vi "GetErrorsOfLibrary.vi"(8 "ErrorIn":errorcluster caption="Error In(no Error)", 9 "LibraryName":string, 11 "ReferenceIn":refnum<class "ErrorDefinitionSQLite.lvclass"> caption="Reference In") -> (0 "ErrorOut":errorcluster caption="Error Out", 1 "Errors":T1, 3 "ReferenceOut":refnum<class "ErrorDefinitionSQLite.lvclass"> caption="Reference Out")   [LabVIEW 2018, in "ErrorDefinitionSQLite.lvclass"]
uses:
  <userlib>/_express/CustomErrorCreator/ErrorDefinitionSQLite/ErrorDefinitionSQLite.lvclass
  <userlib>/_express/CustomErrorCreator/ErrorDefinitionSQLite/ErrorContent.ctl
  <vilib>/drjdpowell/SQLite Library/SQL Connection/Open (path).vi
  <vilib>/drjdpowell/SQLite Library/SQL Connection/Open (string).vi
  <vilib>/AdvancedString/Path To Command Line String.vi
  <vilib>/drjdpowell/SQLite Library/SQL Connection/Execute SQL.vi
  <vilib>/drjdpowell/SQLite Library/SQL Connection/Connection.lvclass
  <vilib>/drjdpowell/SQLite Library/SQLite.lvlib
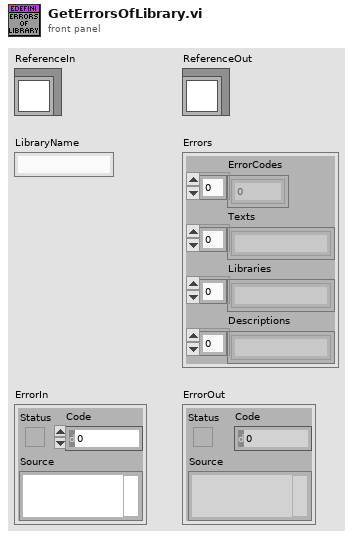
[diagram p1: front panel]
types:
  T1 = typedef "ErrorDefinitionSQLite.lvclass/ErrorContent.ctl" = cluster{"ErrorCodes":i32[], "Texts":string[], "Libraries":string[], "Descriptions":string[]}
  T2 = enum16{"New or existing", "Existing", "Read only"}
  T3 = typedef "ErrorDefinitionSQLite.lvclass/ObjectAttributes.ctl" = cluster{"Path":path}
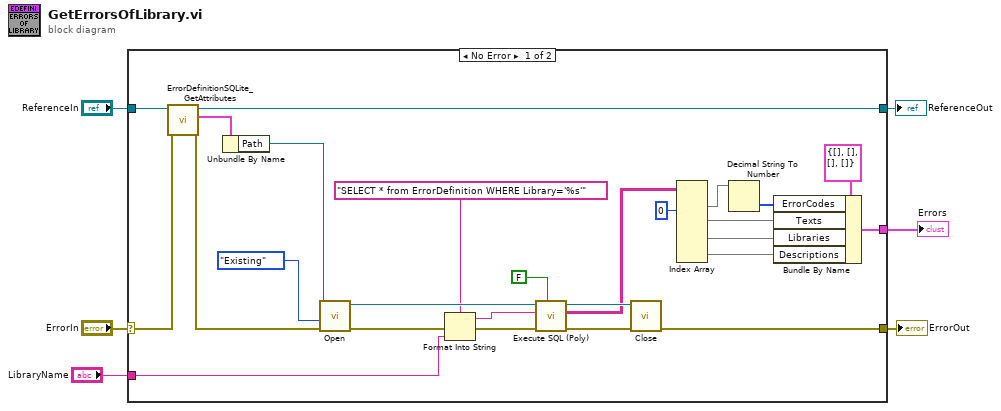
[diagram p0: block diagram]
diagram:
  n1 = case shown="No Error" "ErrorIn" {
    selector: "ErrorIn" -> [w32 w34]
    tunnel: [w16 w34] -> w5
    tunnel: [w30 w33] -> w3
    tunnel: "ReferenceIn" -> [w31 w33]
    tunnel: "LibraryName" -> [w19 _]
    tunnel: [w7 _] -> w1
    frame No Error {
      n2 = call <userlib>:"ErrorDefinitionSQLite_GetAttributes.vi"("ErrorIn"=w32, "Reference in"=w31) -> ("ErrorOut"=w26:errorcluster, "Data"=w28:T3, "Reference out"=w30:refnum<class "ErrorDefinitionSQLite.lvclass">)  [unwired: 6 in, 1 out]
      n3 = Unbundle By Name(w28) -> ("Path"=w27:path)
      n4 = call-poly <vilib>:"Open.vi"("error in (no error)"=w26, "File Option"=T2."Existing", "db file"=w27) -> ("error out"=w21:errorcluster, "SQLite Connection"=w24:refnum<class "Connection.lvclass">)  [unwired: 7 in]
      n5 = Format Into String(format string="SELECT * from ErrorDefinition WHERE Library='%s'" ("SQL"), error in=w21, w19) -> (resulting string=w22:string, error out=w20:errorcluster)  [unwired: 1 in]
      n6 = call-poly <vilib>:"Execute SQL (Poly).vi"("Use SAVEPOINT"=FALSE, "error in (no error)"=w20, "SQL"=w22, "SQLite Connection in"=w24) -> ("error out"=w17:errorcluster, "Result Set"=w15:string[][], "SQLite Connection"=w18:refnum<class "Connection.lvclass">)  [unwired: 4 in, 1 out]
      n7 = call-dynamic "Close.vi"("error in (no error)"=w17, "SQLite Connection in"=w18) -> ("error out"=w16:errorcluster)  [unwired: 9 in]
      n8 = Index Array(array=w15, index (col) #1=0 ("disabled index (col)")) -> (element #1=w9:string[], element #2=w10:string[], element #3=w11:string[], element #4=w12:string[])  [unwired: 7 in]
      n9 = Decimal String To Number(string=w9) -> (number=w8:i32[])  [unwired: 2 in, 1 out]
      n10 = Bundle By Name(cluster=T1 {"ErrorCodes"=[], "Texts"=[], "Libraries"=[], "Descriptions"=[]} ("Errors"), "ErrorCodes"=w8, "Texts"=w10, "Libraries"=w11, "Descriptions"=w12) -> (w7:T1)
    }
    frame Error {
    }
  }
  "ErrorOut" <- w5
  "ReferenceOut" <- w3
  "Errors" <- w1
